vi "Parallel Discover Plugins.vi"(8 "error in (no error)":errorcluster, 10 "Update Metadata":bool, 11 "CIFPluginManager in":refnum<class "CIFPluginManager.lvclass">) -> (0 "error out":errorcluster, 3 "CIFPluginManager out":refnum<class "CIFPluginManager.lvclass">)   [LabVIEW 2021, in "CIFPluginManager.lvclass"]
uses:
  CIFPluginManager.lvclass
  CIFPluginManager.lvclass/CIFPluginManager.ctl
  CIFCore/Common/Typedef/Version.ctl
  CIFCore/Common/CIFCoreCommon.lvlib
  typedef/Discovered Plugin.ctl
  typedef/Plugin Metadata.ctl
  typedef/Loader Type.ctl
  <vilib>/Utility/LVLibp/NI_PackedLibraryUtility.lvlib
  CIFUtilities/CIFConfigurationFile/CIF Configuration File.lvlib
  CIFUtilities/CIFConfigurationFile/typedef/Location Type.ctl
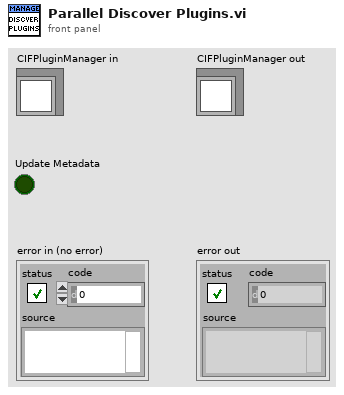
[diagram p1: front panel]
types:
  T1 = typedef "CIF Configuration File.lvlib/Location Type.ctl" = enum16{"Config File", "Manager", "Protos", "Plugins", "UI Plugins", "Logs", "Orchestrations"}
  T2 = typedef "CIFPluginManager.lvclass/Discovered Plugin.ctl" = cluster{"Filename":string, "Plugin Type":string, "Qualified name":string, "Version":T3, "Plugin Metadata":T4, "Launcher":T5, "File Path":string}
  T3 = typedef "CIFCoreCommon.lvlib/Version.ctl" = cluster{"Major":i32, "Minor":i32, "Fix":i32, "Build":i32}
  T4 = typedef "CIFPluginManager.lvclass/Plugin Metadata.ctl" = cluster{"Description":string, "History":string, "Author":string}
  T5 = typedef "CIFPluginManager.lvclass/Loader Type.ctl" = enum16{"LabVIEW"}
  T6 = typedef "CIFPluginManager.lvclass/Discovered Plugin Map.ctl" = map{string, T2[]}
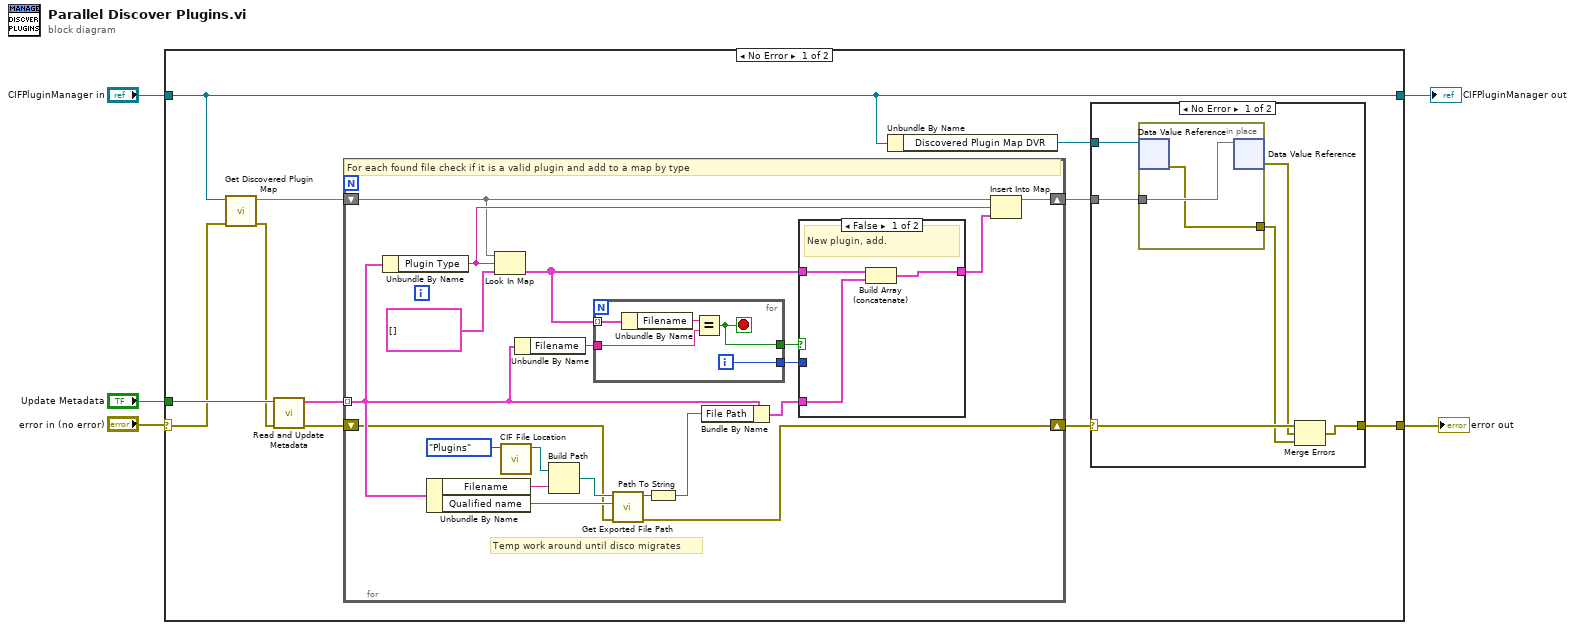
[diagram p0: block diagram]
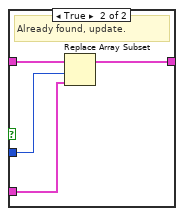
[diagram p3: hidden frame]
diagram:
  n1 = case shown="No Error" "error in (no error)" {
    selector: "error in (no error)" -> [w12 w58]
    tunnel: "CIFPluginManager in" -> [w10 w59]
    tunnel: [w10 w59] -> w3
    tunnel: [w8 w58] -> w5
    tunnel: "Update Metadata" -> [w16 _]
    frame No Error {
      n2 = call "Get Discovered Plugin Map.vi"("error in (no error)"=w12, "CIFPluginManager in"=w10) -> ("error out"=w11:errorcluster, "Discovered Plugins"=w13:T6)  [unwired: 8 in]
      n3 = call "Read and Update Metadata.vi"("error in (no error)"=w11, "Update Metadata"=w16) -> ("error out"=w15:errorcluster, "Plugin Info"=w14:T2[])  [unwired: 8 in]
      n4 = for {
        shift-right: [w26] -> w9
        shift-left: w15 -> [w27]
        tunnel: w14 -> [w31] mode=indexing
        shift-right: [w37] -> w6
        shift-left: w13 -> [w38]
        # "Temp work around until disco migrates"
        # "For each found file check if it is a valid plugin and add to a map by type"
        n5 = Unbundle By Name(w31) -> ("Plugin Type"=w39:string)
        n6 = Unbundle By Name(w31) -> ("Filename"=w35:string, "Qualified name"=w34:string)
        n7 = Look In Map(map=w38, key=w39, default value=T2[] [] ("value")) -> (value=w42:T2[])  [unwired: 1 out]
        n8 = call "CIF File Location.vi"("LocationType"=Location_Type."Plugins") -> ("Location"=w32:path)  [unwired: 10 in]
        n9 = Unbundle By Name(w31) -> ("Filename"=w44:string)
        n10 = Build Path(base path=w32, name or relative path=w35) -> (appended path=w36:path)
        n11 = for {
          tunnel: w44 -> [w56]
          tunnel: w42 -> [w53] mode=indexing
          tunnel: [w55] -> w43
          tunnel: [w54] -> w41
          i -> [w54]
          stop <- w55 stop-if-true
          n12 = Unbundle By Name(w53) -> ("Filename"=w57:string)
          n13 = Equal?(x=w57, y=w56) -> (x = y?=w55:bool)
        }
        n14 = call <vilib>:"Get Exported File Path.vi"("error in (no error)"=w27, "qualified name"=w34, "packed library path"=w36) -> ("error out"=w26:errorcluster, "path"=w30:path)  [unwired: 7 in]
        n15 = Path To String(path=w30) -> (string=w29:string)
        n16 = Bundle By Name(cluster=w31, "File Path"=w29) -> (w28:T2)
        n17 = case shown="False" w43 {
          tunnel: w28 -> [w47 w52]
          tunnel: w42 -> [w48 w51]
          tunnel: [w46 w49] -> w40
          tunnel: w41 -> [_ w50]
          frame False {
            # "New plugin, add."
            n18 = Build Array (concatenate)(w48, w47) -> (w46:T2[])
          }
          frame True {
            # "Already found, update."
            n19 = Replace Array Subset(array=w51, new element=w52, index=w50) -> (w49:T2[])
          }
        }
        n20 = Insert Into Map(map in=w38, key=w39, value=w40) -> (map out=w37:T6)  [unwired: 2 out]
      }
      n21 = Unbundle By Name(w10) -> ("Discovered Plugin Map DVR"=w7:refnum<data-value>)
      n22 = case shown="No Error" w9 {
        selector: w9 -> [w20 w25]
        tunnel: [w17 w25] -> w8
        tunnel: w7 -> [w22 _]
        tunnel: w6 -> [w21 _]
        frame No Error {
          n23 = in-place {
            in-place-border: w21 -> [w24]
            in-place-border: [w23] -> w18
            n24 = in-place-dvr #1(w22) -> (w23:errorcluster)  [unwired: 1 out]
            n25 = in-place-dvr #1(w24) -> (w19:errorcluster)  [unwired: 1 out]
          }
          n26 = Merge Errors(w20, w19, w18) -> (w17:errorcluster)
        }
        frame Error {
        }
      }
    }
    frame Error {
    }
  }
  "error out" <- w5
  "CIFPluginManager out" <- w3
